vi "Create Reference Enqueuer.vi"(6 "Name":string, 8 "error in":errorcluster, 10 "Timeout (s)":i32=10) -> (0 "error out":errorcluster, 3 "QDMH out":refnum<class "QDMH.lvclass">)   [LabVIEW 2023, in "QDMH.lvlib" / "QDMH.lvclass"]
doc: "This defines the unique name of the message queue spawned. It is required if a VI reference is not passed into this VI.\n\nThis defines the program named queue handle. If the caller VI passes its reference to this VI, the queue will take on the name of the caller VI. \n\n**Caution** using the caller VI name will not generate unique queue handles so it should only be used for top level applications that are not spawned as multiple instances."
uses:
  QDMH.lvclass
  Custom Controls/QDMH Message.ctl
  QDMH.lvclass/QDMH.ctl
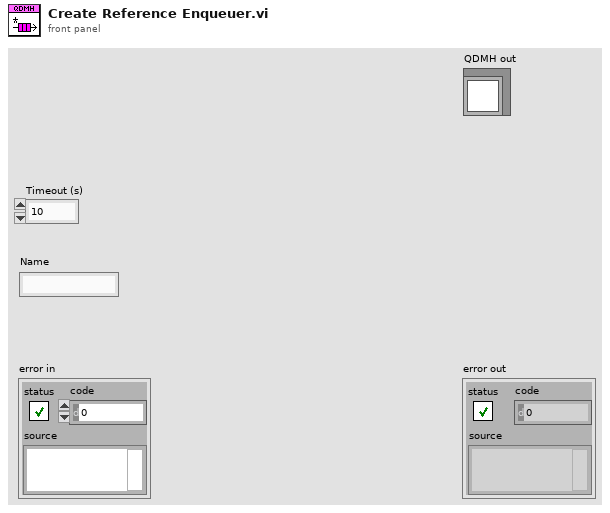
[diagram p1: front panel]
types:
  T1 = typedef "QDMH.lvlib/QDMH.lvclass/QDMH Message.ctl" = cluster{"State":string, "Data":variant}
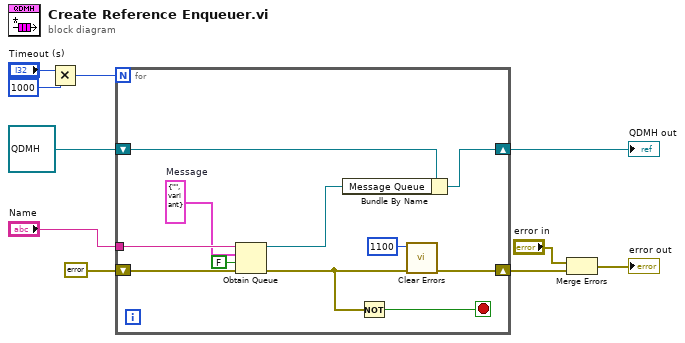
[diagram p0: block diagram]
diagram:
  n1 = Multiply(x="Timeout (s)", y=1000) -> (x*y=w5:i32)
  n2 = for {
    N: w5 -> [_]
    tunnel: "Name" -> [w18]
    shift-right: [w20] -> w8
    shift-left: refnum<class "QDMH.lvclass"> refnum ("QDMH in") -> [w21]
    shift-right: [w12] -> w10
    shift-left: errorcluster {"status"=FALSE, "code"=0, "source"=""} ("error out") -> [w19]
    stop <- w13 stop-if-true
    w17 = T1 {"State"="", "Data"=variant}  # Message
    n3 = Obtain Queue(name (unnamed)=w18, element data type=w17, create if not found? (T)=FALSE, error in (no error)=w19) -> (queue out=w16:refnum<queue>, error out=w14:errorcluster)  [unwired: 1 in, 1 out]
    n4 = Bundle By Name(cluster=w21, "Message Queue"=w16) -> (w20:refnum<class "QDMH.lvclass">)
    n5 = Not(x=w14) -> (.not. x?=w13:bool)
    n6 = call <vilib>:"Clear Errors.vi"("error in (no error)"=w14, "specific error code to clear (0: all)"=1100) -> ("error out"=w12:errorcluster)  [unwired: 4 in, 1 out]
  }
  "QDMH out" <- w8
  n7 = Merge Errors("error in", w10) -> (→"error out":errorcluster)
